vi "AT Create Buffer A.vi"(8 "error in (no error)":errorcluster, 9 "Buffer":u64, 10 "Size":i32, 11 "Handle":i32) -> (0 "error out":errorcluster, 2 "Buffer out":u64, 3 "Status":i32)   [LabVIEW 2019]
doc: "CreateBuffer\n\nOutput:\n I32 Status\n U64 Buffer out\n\nInput:\n I32 Handle\n I32 Size\n U64 Buffer\n\nCreates and allocates memory for an instance of a buffer."
uses:
  atcoreA.dll
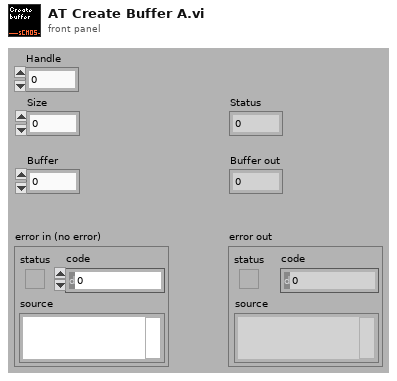
[diagram p1: front panel]
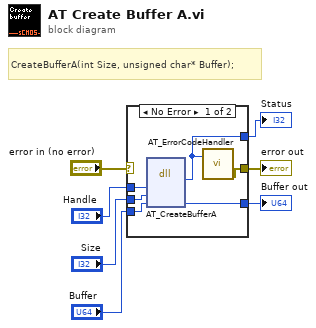
[diagram p0: block diagram]
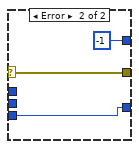
[diagram p2: hidden frame]
diagram:
  # "CreateBufferA(int Size, unsigned char* Buffer);"
  n1 = case shown="No Error" "error in (no error)" {
    selector: "error in (no error)" -> [_ w16]
    tunnel: [w9 w16] -> w6
    tunnel: [w8 -1] -> w5
    tunnel: [w13 w14] -> w4
    tunnel: "Buffer" -> [w12 w14]
    tunnel: "Size" -> [w11 _]
    tunnel: "Handle" -> [w10 _]
    frame No Error {
      n2 = dll-call lib="atcoreA.dll" fn="AT_CreateBufferA"("Handle"=w10, "Size"=w11, "Buffer"=w12) -> ("Status"=w8:i32, "Buffer"=w13:u64)  [unwired: 5 in, 2 out]
      n3 = call <userlib>:"AT_ErrorCodeHandler.vi"("Error"=w8) -> ("error out"=w9:errorcluster)  [unwired: 6 in]
    }
    frame Error {
    }
  }
  "Status" <- w5
  "Buffer out" <- w4
  "error out" <- w6
